vi "main.vi"() -> ()   [LabVIEW 2018]
uses:
  controls/Button Previous.ctl
  controls/Button Next.ctl
  support/classes/MonthDisplay/month.ctl
  support/classes/Banking Statement/BankingTransactionList.lvclass
  C:/GitRepos/Filthy-Lucre-Budgetizer/source/support/classes/Statement/TransactionList.lvclass
  support/classes/Credit Statement/CreditTransactionList.lvclass
  support/classes/Goal/Goal.lvclass
  C:/GitRepos/Filthy-Lucre-Budgetizer/source/support/classes/UserEditableAmount/UserEditableAmount.lvclass
  support/classes/TransactionListUserInterface/TransactionListUIAdapter.lvclass
  support/classes/database/Account History.lvclass
  support/classes/UserEditableAmount/UserEditableAmount.lvclass
  support/classes/Category/Category.lvclass
  support/classes/MonthDisplay/DateUserInterface.lvclass
  support/classes/GoalUserInterface/OutcomeListUIAdapter.lvclass
panel:
  in  "Month":T1
  in  "Tab Control":enum32{"Summary", "Banking", "Credit", "Report"}(tab)
  in  "Delete Goal":bool
  in  "Edit Goal":bool
  in  "Summary":i32(listbox)
  out "Banking":i32(listbox)
  in  "Credit":i32[](listbox)
  out "Balance":dbl format="%.2f"
  in  "Next":T2
  in  "Prev":T3
  in  "Year":i32=2008
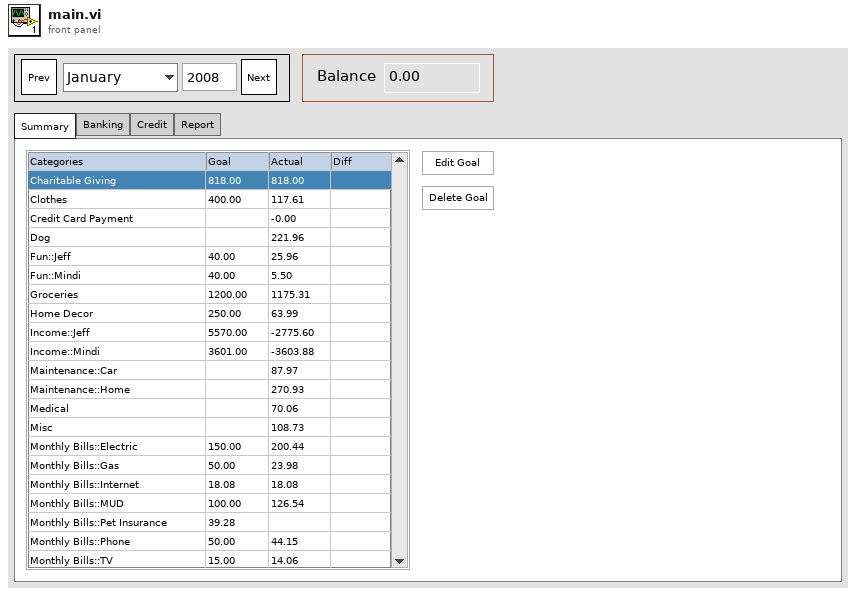
[diagram p1: front panel]
types:
  T1 = typedef "DateUserInterface.lvclass/month.ctl" = enum16{"January", "February", "March", "April", "May", "June", "July", "August", "September", "October", "November", "December"}
  T2 = typedef "Button Next.ctl" = bool
  T3 = typedef "Button Previous.ctl" = bool
  T4 = enum8{"Enabled", "Disabled", "Disabled and Grayed Out"}
  T5 = typedef "LVPoint32TypeDef.ctl" = cluster{"Horizontal":i32, "Vertical":i32}
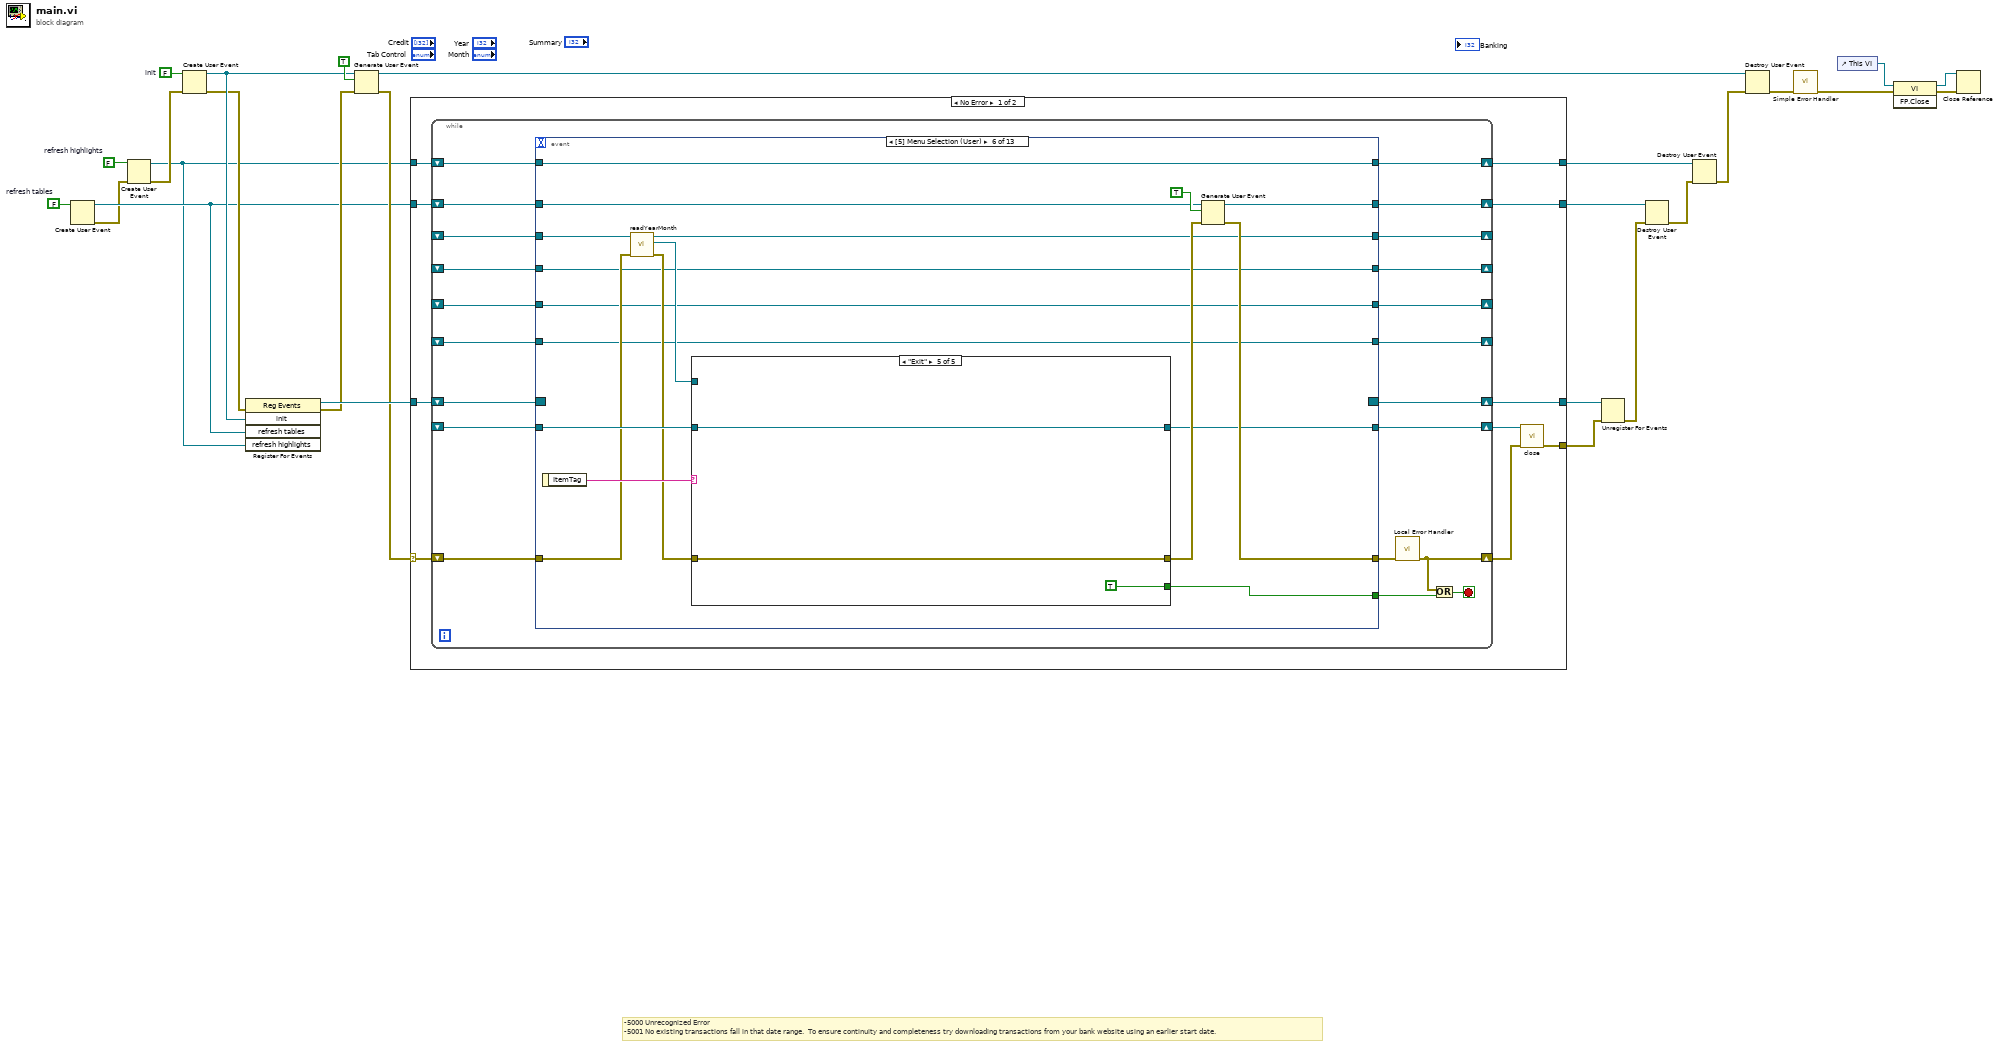
[diagram p0: block diagram]
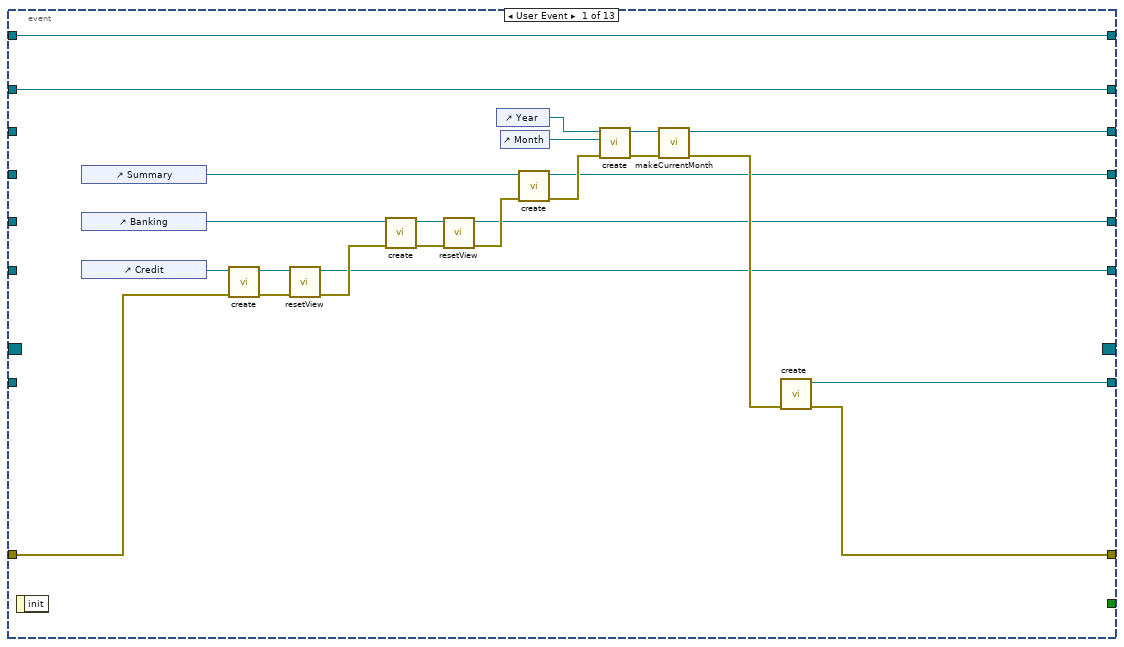
[diagram p2: hidden frame]
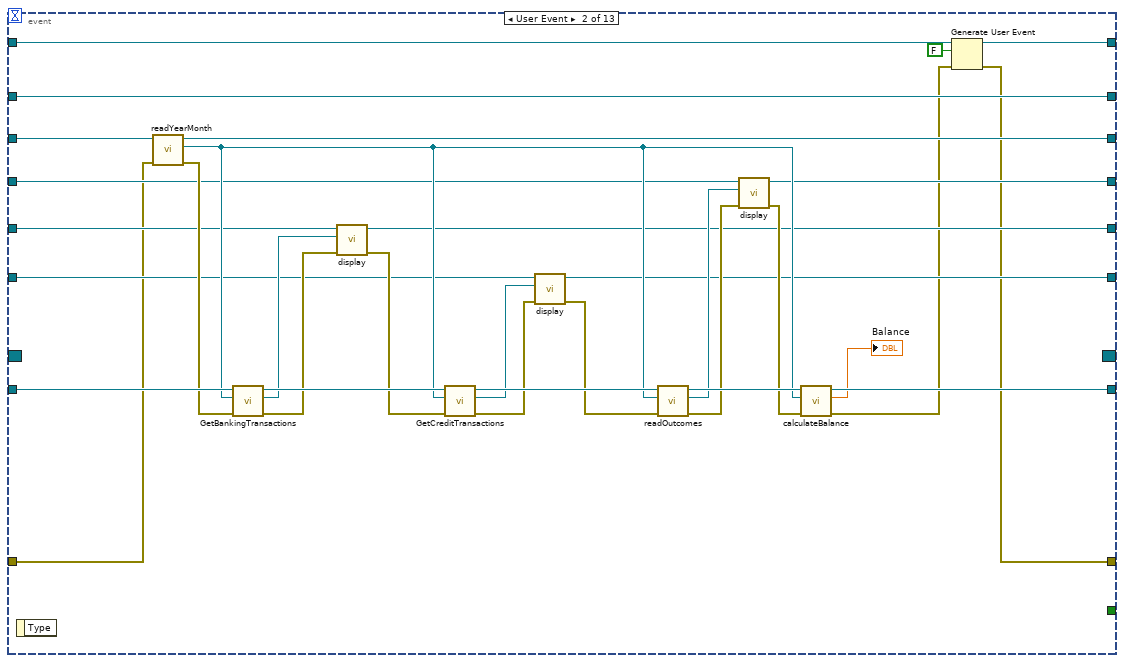
[diagram p3: hidden frame]
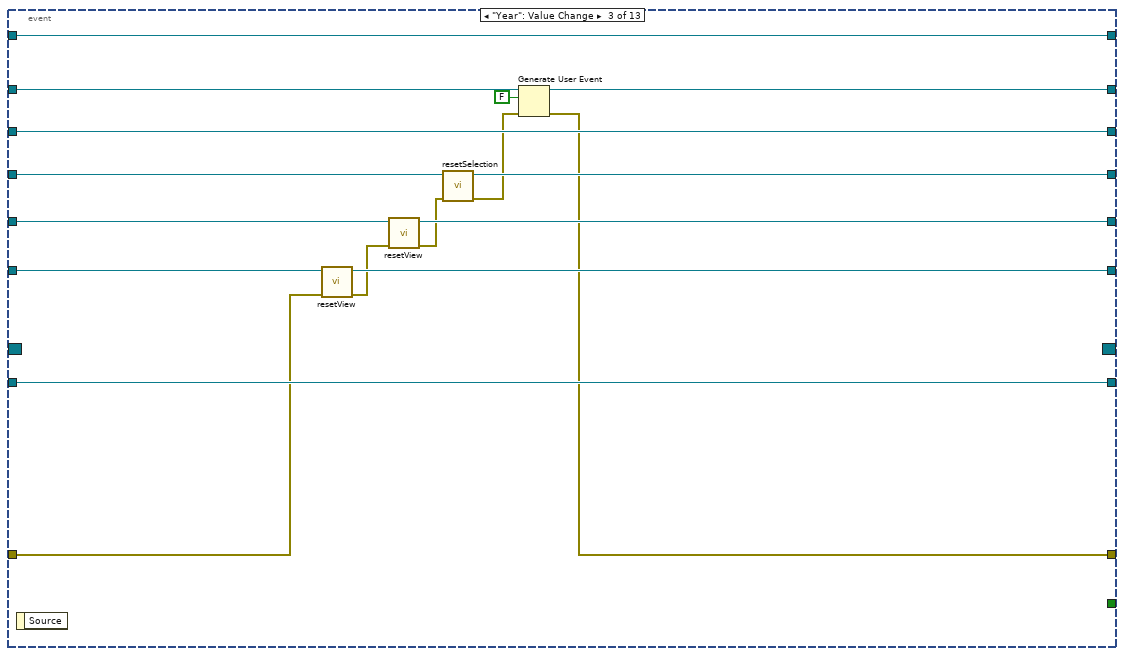
[diagram p4: hidden frame]
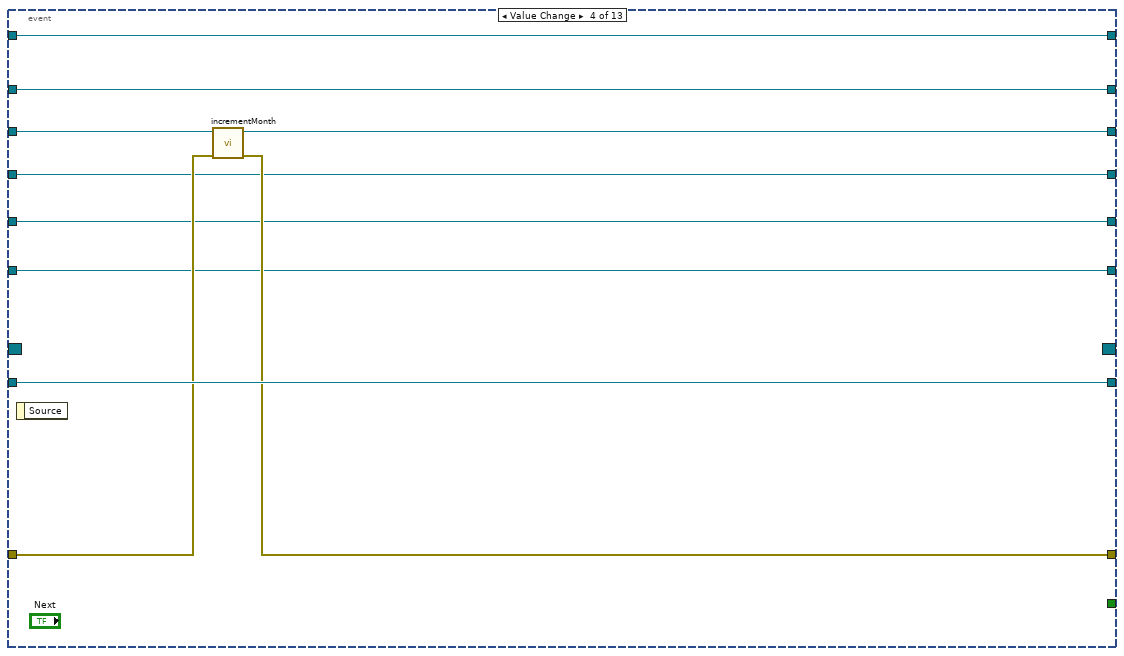
[diagram p5: hidden frame]
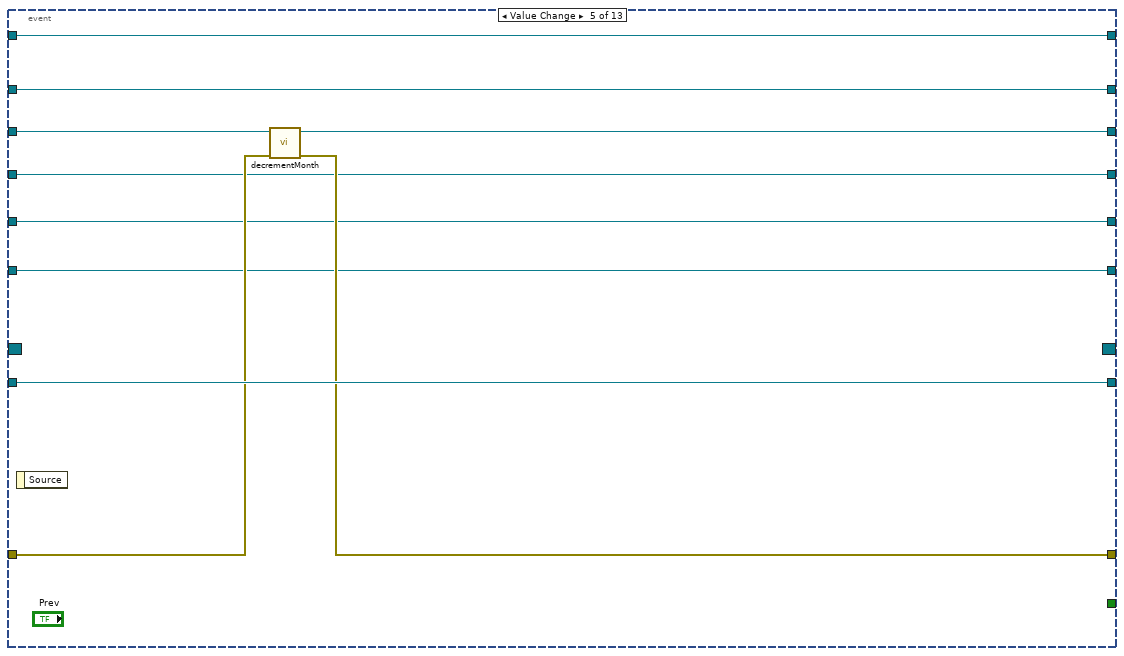
[diagram p6: hidden frame]
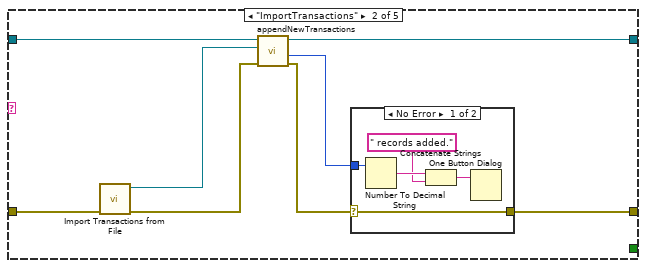
[diagram p8: hidden frame]
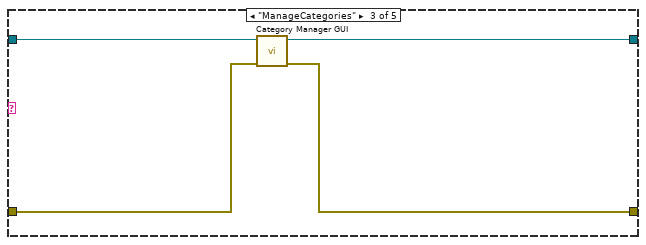
[diagram p10: hidden frame]
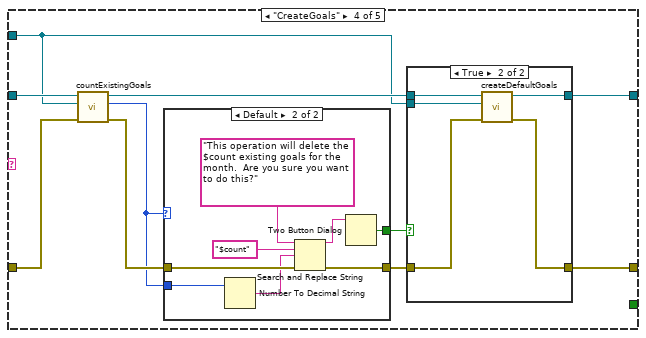
[diagram p11: hidden frame]
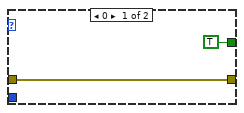
[diagram p12: hidden frame]
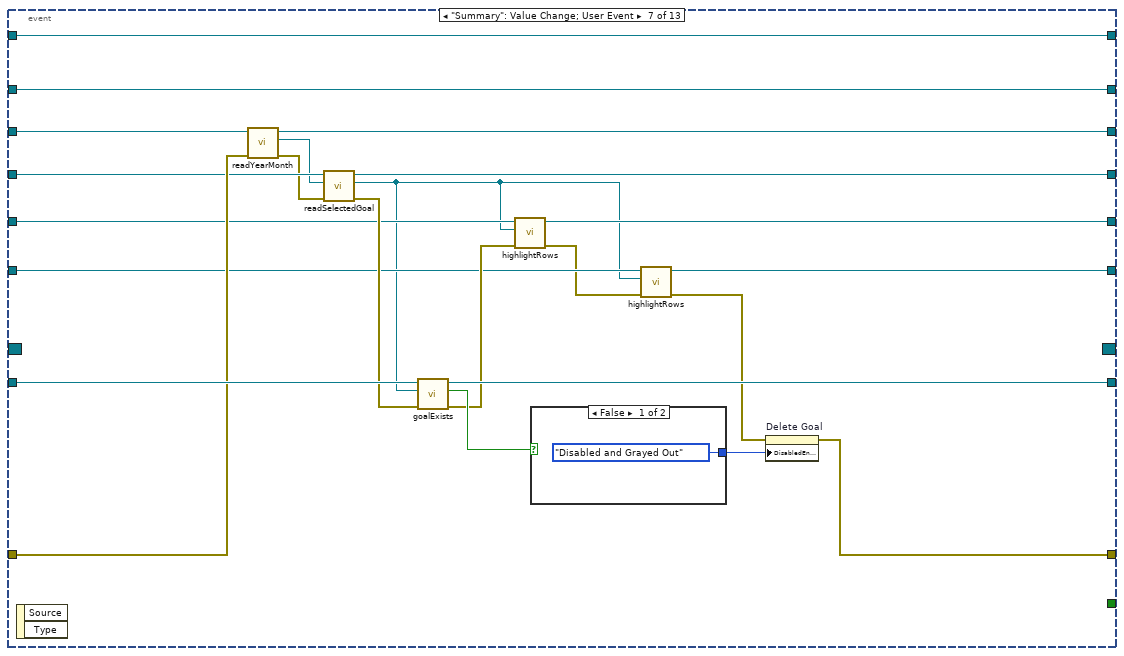
[diagram p14: hidden frame]
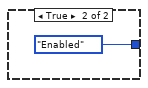
[diagram p15: hidden frame]
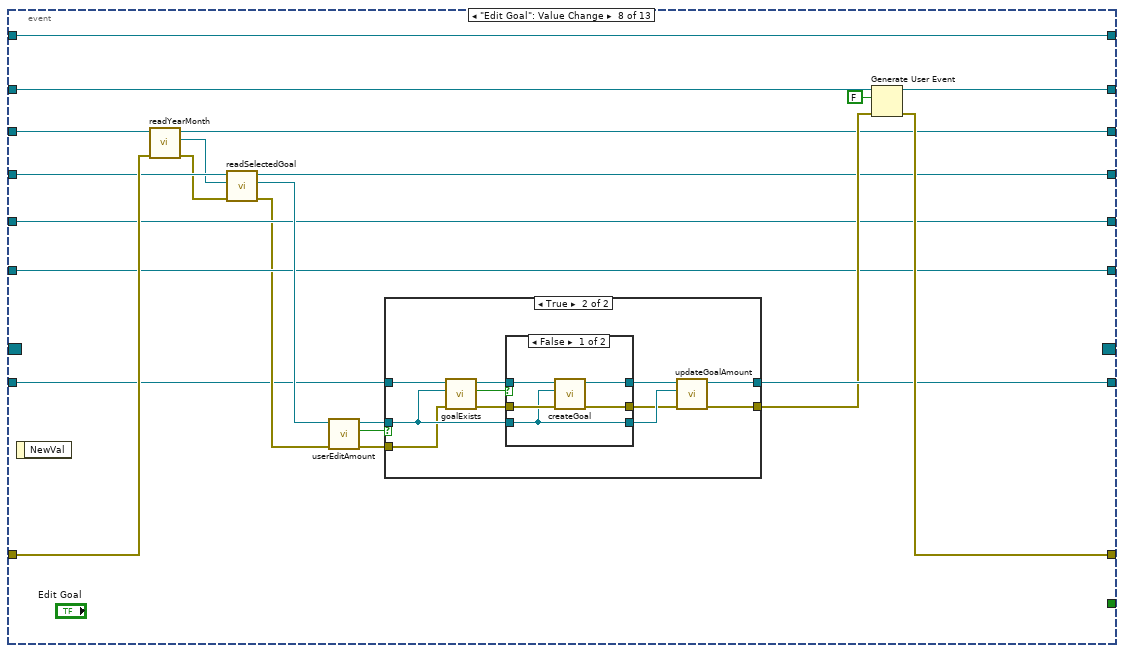
[diagram p16: hidden frame]
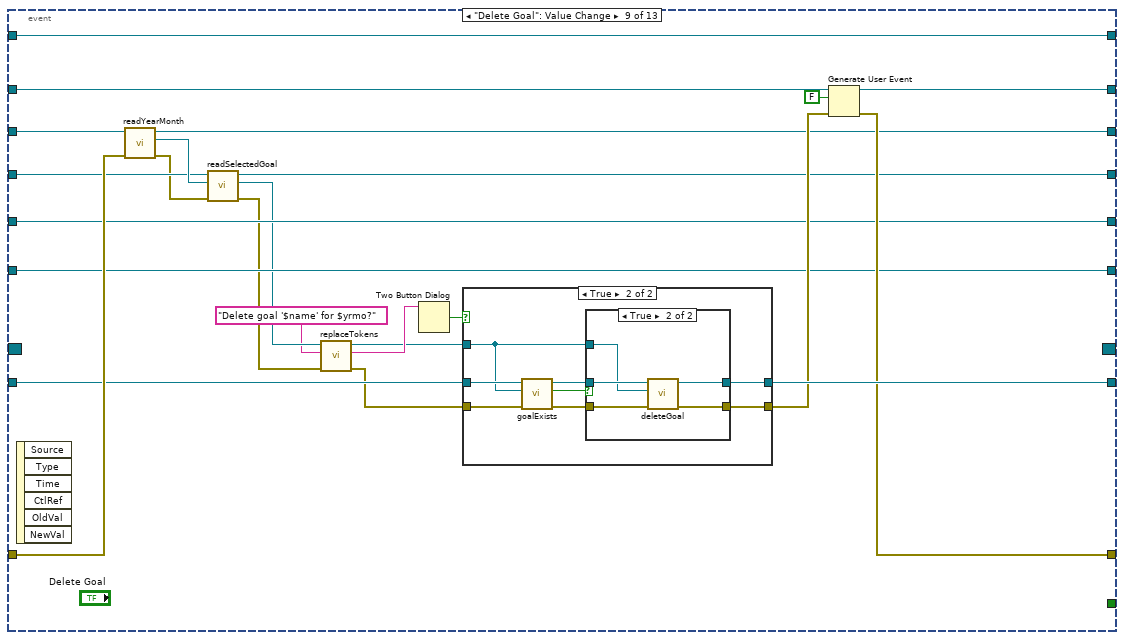
[diagram p19: hidden frame]
diagram:
  w5 = FALSE  # refresh highlights
  w15 = FALSE  # refresh tables
  w24 = FALSE  # init
  # "-5000 Unrecognized Error\n-5001 No existing transactions fall in that date range.  To ensure continuity and completeness try downloading transactions from your bank website using an earlier start date."
  n1 = Create User Event(user event datatype=w15) -> (user event=w14:refnum<user-event>, error out=w7:errorcluster)  [unwired: 1 in]
  n2 = Create User Event(user event datatype=w5, error in=w7) -> (user event=w4:refnum<user-event>, error out=w6:errorcluster)
  n3 = Create User Event(user event datatype=w24, error in=w6) -> (user event=w21:refnum<user-event>, error out=w17:errorcluster)
  n4 = register-events(error in=w17, w21, w14, w4) -> (reference out=w26:refnum<event-registration>, error out=w20:errorcluster)  [unwired: 1 in]
  n5 = Generate User Event(user event=w21, event data cluster=TRUE ("event data"), error in=w20) -> (user event out=w18:refnum<user-event>, error out=w19:errorcluster)  [unwired: 1 in]
  n6 = case shown="No Error" w19 {
    selector: w19 -> [w34 w396]
    tunnel: w26 -> [w36 w397]
    tunnel: [w29 w396] -> w16
    tunnel: [w35 w397] -> w25
    tunnel: w14 -> [w33 w395]
    tunnel: [w32 w395] -> w13
    tunnel: w4 -> [w28 w394]
    tunnel: [w27 w394] -> w3
    frame No Error {
      n7 = while {
        shift-right: [w53] -> w30
        shift-left: w34 -> [w56]
        shift-right: [w55] -> w35
        shift-left: w36 -> [w57]
        shift-right: [w49] -> w31
        shift-left: _ -> [w50]
        shift-right: [w47] -> w32
        shift-left: w33 -> [w48]
        shift-right: [w46] -> _
        shift-left: _ -> [w43]
        shift-right: [w45] -> _
        shift-left: _ -> [w44]
        shift-right: [w42] -> _
        shift-left: _ -> [w41]
        shift-right: [w40] -> _
        shift-left: _ -> [w39]
        shift-right: [w37] -> w27
        shift-left: w28 -> [w38]
        stop <- w52 stop-if-true
        n8 = event shown="[5] Menu Selection (User)" {
          selector: w57 -> [_ _ _ _ _ _ _ _ _ _ _ _ _]
          dyn-events: [_ _ _ _ _ _ _ _ _ _ _ _ _] -> w55
          timeout: _ -> [_ _ _ _ _ _ _ _ _ _ _ _ _]
          tunnel: w56 -> [w67 w87 w119 w137 w146 w157 w234 w258 w304 w335 w356 w366 w393]
          tunnel: [w79 w83 w114 w135 w145 w163 w238 w263 w307 w346 w355 w382 w393] -> w54
          tunnel: [_ _ _ _ _ w151 _ _ _ _ _ _ w386] -> w51
          tunnel: w50 -> [_ w112 w128 w140 w150 w167 w240 w244 w302 w341 w360 w380 w391]
          tunnel: [w81 w111 w128 w140 w150 w161 w239 w262 w310 w341 w359 w379 w391] -> w49
          tunnel: w48 -> [w80 w113 w130 w139 w149 w165 w241 w265 w308 w342 w354 w383 w392]
          tunnel: [w80 w113 w129 w139 w149 w164 w241 w264 w309 w342 w354 w384 w392] -> w47
          tunnel: [w75 w106 w127 w136 w147 w159 w233 w259 w303 w332 w352 w377 w390] -> w46
          tunnel: w43 -> [_ w107 w127 w138 w148 w160 w235 w260 w305 w332 w352 w377 w390]
          tunnel: [w70 w99 w121 w134 w144 w155 w231 w251 w298 w331 w351 w376 w389] -> w45
          tunnel: w44 -> [_ w88 w120 w134 w144 w155 w232 w254 w300 w331 w351 w376 w389]
          tunnel: [w62 w98 w123 w133 w143 w154 w225 w249 w296 w330 w350 w374 w388] -> w42
          tunnel: w41 -> [_ w90 w125 w133 w143 w154 w227 w249 w296 w330 w350 w374 w388]
          tunnel: [w58 w91 w122 w132 w142 w153 w221 w248 w297 w329 w349 w373 w387] -> w40
          tunnel: w39 -> [_ w89 w124 w132 w142 w153 w224 w248 w297 w329 w349 w373 w387]
          tunnel: w38 -> [w66 w86 w115 w131 w141 w152 w219 w246 w294 w328 w348 w363 w385]
          tunnel: [w66 w85 w115 w131 w141 w152 w219 w246 w294 w328 w348 w363 w385] -> w37
          event User Event {
            n9 = event-data() -> ()  [unwired: 1 in, 1 out]
            n10 = control-ref of="Summary"() -> (w73:refnum<vi>)
            n11 = control-ref of="Banking"() -> (w69:refnum<vi>)
            n12 = control-ref of="Credit"() -> (w68:refnum<vi>)
            n13 = call "create.vi"("error in (no error)"=w67, "MulticolumnListbox in"=w68) -> ("error out"=w61:errorcluster, "TransactionListUserInterface out"=w60:refnum<class "TransactionListUIAdapter.lvclass">)  [unwired: 8 in]
            n14 = call-dynamic "resetView.vi"("error in (no error)"=w61, "TransactionListUserInterface in"=w60) -> ("error out"=w59:errorcluster, "TransactionListUserInterface out"=w58:refnum<class "TransactionListUIAdapter.lvclass">)  [unwired: 8 in]
            n15 = call "create.vi"("error in (no error)"=w59, "MulticolumnListbox in"=w69) -> ("error out"=w64:errorcluster, "TransactionListUserInterface out"=w65:refnum<class "TransactionListUIAdapter.lvclass">)  [unwired: 8 in]
            n16 = call-dynamic "resetView.vi"("error in (no error)"=w64, "TransactionListUserInterface in"=w65) -> ("error out"=w63:errorcluster, "TransactionListUserInterface out"=w62:refnum<class "TransactionListUIAdapter.lvclass">)  [unwired: 8 in]
            n17 = control-ref of="Year"() -> (w78:refnum<vi>)
            n18 = control-ref of="Month"() -> (w77:refnum<vi>)
            n19 = call "create.vi"("error in (no error)"=w63, "Summary"=w73) -> ("error out"=w71:errorcluster, "GoalUserInterface out"=w70:refnum<class "OutcomeListUIAdapter.lvclass">)  [unwired: 8 in]
            n20 = call "create.vi"("error in (no error)"=w71, "Month"=w77, "Year"=w78) -> ("error out"=w74:errorcluster, "MonthDisplay out"=w76:refnum<class "DateUserInterface.lvclass">)  [unwired: 7 in]
            n21 = call "makeCurrentMonth.vi"("error in (no error)"=w74, "MonthDisplay in"=w76) -> ("error out"=w72:errorcluster, "MonthDisplay out"=w75:refnum<class "DateUserInterface.lvclass">)  [unwired: 8 in]
            n22 = call "create.vi"("error in (no error)"=w72) -> ("error out"=w79:errorcluster, "Database.lvclass"=w81:refnum<class "Account History.lvclass">)  [unwired: 9 in]
          }
          event User Event {
            n23 = event-data() -> ()  [unwired: 1 in, 1 out]
            n24 = call "readYearMonth.vi"("error in (no error)"=w87, "MonthDisplay in"=w107) -> ("error out"=w104:errorcluster, "WhichMonth.lvclass"=w105:refnum<class "WhichMonth.lvclass">, "MonthDisplay out"=w106:refnum<class "DateUserInterface.lvclass">)  [unwired: 7 in]
            n25 = call "GetBankingTransactions.vi"("error in (no error)"=w104, "WhichMonth"=w105, "Database in"=w112) -> ("error out"=w96:errorcluster, "Banking Transactions out"=w97:refnum<class "BankingTransactionList.lvclass">, "Database out"=w109:refnum<class "Account History.lvclass">)  [unwired: 6 in]
            n26 = call "display.vi"("error in (no error)"=w96, "TransactionList.lvclass"=w97, "TransactionListUserInterface in"=w90) -> ("error out"=w95:errorcluster, "TransactionListUserInterface out"=w98:refnum<class "TransactionListUIAdapter.lvclass">)  [unwired: 7 in]
            n27 = call "GetCreditTransactions.vi"("error in (no error)"=w95, "WhichMonth"=w105, "Account History in"=w109) -> ("error out"=w93:errorcluster, "Credit Transactions out"=w94:refnum<class "CreditTransactionList.lvclass">, "Account History out"=w108:refnum<class "Account History.lvclass">)  [unwired: 6 in]
            n28 = call "display.vi"("error in (no error)"=w93, "TransactionList.lvclass"=w94, "TransactionListUserInterface in"=w89) -> ("error out"=w92:errorcluster, "TransactionListUserInterface out"=w91:refnum<class "TransactionListUIAdapter.lvclass">)  [unwired: 7 in]
            n29 = call "readOutcomes.vi"("error in (no error)"=w92, "WhichMonth"=w105, "Database in"=w108) -> ("error out"=w102:errorcluster, "OutcomeList.lvclass"=w103:refnum<class "OutcomeList.lvclass">, "Database out"=w110:refnum<class "Account History.lvclass">)  [unwired: 6 in]
            n30 = call "display.vi"("error in (no error)"=w102, "OutcomeList.lvclass"=w103, "GoalUserInterface in"=w88) -> ("error out"=w101:errorcluster, "GoalUserInterface out"=w99:refnum<class "OutcomeListUIAdapter.lvclass">)  [unwired: 7 in]
            n31 = call "calculateBalance.vi"("error in (no error)"=w101, "WhichMonth"=w105, "Database in"=w110) -> ("error out"=w84:errorcluster, "Month Balance"=→"Balance":dbl, "Database out"=w111:refnum<class "Account History.lvclass">)  [unwired: 6 in]
            n32 = Generate User Event(user event=w86, event data cluster=FALSE ("event data"), error in=w84) -> (user event out=w85:refnum<user-event>, error out=w83:errorcluster)  [unwired: 1 in]
          }
          event "Year": Value Change {
            n33 = event-data() -> ()  [unwired: 1 in, 1 out]
            n34 = call-dynamic "resetView.vi"("error in (no error)"=w119, "TransactionListUserInterface in"=w124) -> ("error out"=w118:errorcluster, "TransactionListUserInterface out"=w122:refnum<class "TransactionListUIAdapter.lvclass">)  [unwired: 8 in]
            n35 = call-dynamic "resetView.vi"("error in (no error)"=w118, "TransactionListUserInterface in"=w125) -> ("error out"=w117:errorcluster, "TransactionListUserInterface out"=w123:refnum<class "TransactionListUIAdapter.lvclass">)  [unwired: 8 in]
            n36 = call "resetSelection.vi"("error in (no error)"=w117, "GoalUserInterface in"=w120) -> ("error out"=w116:errorcluster, "GoalUserInterface out"=w121:refnum<class "OutcomeListUIAdapter.lvclass">)  [unwired: 8 in]
            n37 = Generate User Event(user event=w130, event data cluster=FALSE ("event data"), error in=w116) -> (user event out=w129:refnum<user-event>, error out=w114:errorcluster)  [unwired: 1 in]
          }
          event Value Change {
            n38 = event-data() -> ()  [unwired: 1 in, 1 out]
            n39 = call "incrementMonth.vi"("error in (no error)"=w137, "MonthDisplay in"=w138) -> ("error out"=w135:errorcluster, "MonthDisplay out"=w136:refnum<class "DateUserInterface.lvclass">)  [unwired: 8 in]
          }
          event Value Change {
            n40 = event-data() -> ()  [unwired: 1 in, 1 out]
            n41 = call "decrementMonth.vi"("error in (no error)"=w146, "MonthDisplay in"=w148) -> ("error out"=w145:errorcluster, "MonthDisplay out"=w147:refnum<class "DateUserInterface.lvclass">)  [unwired: 8 in]
          }
          event Menu Selection (User) {
            n42 = event-data() -> ("ItemTag"=w168:string)  [unwired: 1 in]
            n43 = call "readYearMonth.vi"("error in (no error)"=w157, "MonthDisplay in"=w160) -> ("error out"=w156:errorcluster, "WhichMonth.lvclass"=w158:refnum<class "WhichMonth.lvclass">, "MonthDisplay out"=w159:refnum<class "DateUserInterface.lvclass">)  [unwired: 7 in]
            n44 = case shown="\"Exit\"" w168 {
              tunnel: w156 -> [w170 w178 w186 w193 w217]
              tunnel: [w170 w174 w185 w197 w217] -> w162
              tunnel: w167 -> [w169 w177 w188 w196 w218]
              tunnel: [w169 w176 w187 w198 w218] -> w161
              tunnel: w158 -> [_ _ _ w194 _]
              tunnel: [_ _ _ _ TRUE] -> w151
              frame Default {
              }
              frame "ImportTransactions" {
                n45 = call "Import Transactions from File.vi"("error in (no error)"=w178) -> ("error out"=w173:errorcluster, "Importing Statement"=w172:refnum<class "TransactionList.lvclass">)  [unwired: 9 in]
                n46 = call "appendNewTransactions.vi"("error in (no error)"=w173, "TransactionList.lvclass"=w172, "Database in"=w177) -> ("error out"=w175:errorcluster, "Num records"=w171:i32, "Database out"=w176:refnum<class "Account History.lvclass">)  [unwired: 6 in]
                n47 = case shown="No Error" w175 {
                  selector: w175 -> [w180 w184]
                  tunnel: [w180 w184] -> w174
                  tunnel: w171 -> [w179 _]
                  frame No Error {
                    n48 = Number To Decimal String(number=w179) -> (decimal integer string=w182:string)  [unwired: 1 in]
                    n49 = Concatenate Strings(w182, " records added.") -> (w183:string)
                    n50 = One Button Dialog(message=w183) -> ()  [unwired: 1 in, 1 out]
                  }
                  frame Error {
                  }
                }
              }
              frame "ManageCategories" {
                n51 = call "Category Manager GUI.vi"("error in (no error)"=w186, "Database.lvclass"=w188) -> ("error out"=w185:errorcluster, "Database.lvclass"=w187:refnum<class "Account History.lvclass">)  [unwired: 8 in]
              }
              frame "CreateGoals" {
                n52 = call "countExistingGoals.vi"("error in (no error)"=w193, "WhichMonth.lvclass"=w194, "Account History in"=w196) -> ("error out"=w192:errorcluster, "Goal  Count"=w189:i32, "Account History out"=w195:refnum<class "Account History.lvclass">)  [unwired: 6 in]
                n53 = case shown="Default" w189 {
                  tunnel: w192 -> [w200 w208]
                  tunnel: w189 -> [_ w207]
                  tunnel: [TRUE ("T button?") w206] -> w191
                  tunnel: [w200 w205] -> w190
                  frame 0 {
                  }
                  frame Default {
                    n54 = Number To Decimal String(number=w207) -> (decimal integer string=w201:string)  [unwired: 1 in]
                    n55 = Search and Replace String(input string="This operation will delete the $count existing goals for the month.  Are you sure you want to do this?", search string="$count", replace string=w201, error in=w208) -> (result string=w204:string, error out=w205:errorcluster)  [unwired: 4 in, 2 out]
                    n56 = Two Button Dialog(message=w204) -> (T button?=w206:bool)  [unwired: 2 in]
                  }
                }
                n57 = case shown="True" w191 {
                  tunnel: w195 -> [w210 w215]
                  tunnel: [w210 w214] -> w198
                  tunnel: w190 -> [w209 w213]
                  tunnel: [w209 w212] -> w197
                  tunnel: w194 -> [_ w211]
                  frame False {
                  }
                  frame True {
                    n58 = call "createDefaultGoals.vi"("error in (no error)"=w213, "WhichMonth"=w211, "Database in"=w215) -> ("error out"=w212:errorcluster, "Database out"=w214:refnum<class "Account History.lvclass">)  [unwired: 7 in]
                  }
                }
              }
              frame "Exit" {
              }
            }
            n59 = Generate User Event(user event=w165, event data cluster=TRUE ("event data"), error in=w162) -> (user event out=w164:refnum<user-event>, error out=w163:errorcluster)  [unwired: 1 in]
          }
          event "Summary": Value Change; User Event {
            n60 = event-data() -> ()  [unwired: 1 in, 2 out]
            n61 = call "readYearMonth.vi"("error in (no error)"=w234, "MonthDisplay in"=w235) -> ("error out"=w230:errorcluster, "WhichMonth.lvclass"=w229:refnum<class "WhichMonth.lvclass">, "MonthDisplay out"=w233:refnum<class "DateUserInterface.lvclass">)  [unwired: 7 in]
            n62 = call "readSelectedGoal.vi"("error in (no error)"=w230, "WhichMonth.lvclass"=w229, "GoalUserInterface in"=w232) -> ("error out"=w228:errorcluster, "Goal.lvclass"=w223:refnum<class "Goal.lvclass">, "GoalUserInterface out"=w231:refnum<class "OutcomeListUIAdapter.lvclass">)  [unwired: 6 in]
            n63 = call "goalExists.vi"("error in (no error)"=w228, "Goal.lvclass"=w223, "Account History in"=w240) -> ("error out"=w226:errorcluster, "Exists?"=w237:bool, "Account History out"=w239:refnum<class "Account History.lvclass">)  [unwired: 6 in]
            n64 = call "highlightRows.vi"("error in (no error)"=w226, "Goal.lvclass"=w223, "TransactionListUserInterface in"=w227) -> ("error out"=w222:errorcluster, "TransactionListUserInterface out"=w225:refnum<class "TransactionListUIAdapter.lvclass">)  [unwired: 7 in]
            n65 = case shown="False" w237 {
              tunnel: [T4."Disabled and Grayed Out" ("Disabled") T4."Enabled" ("Disabled")] -> w236
              frame False {
              }
              frame True {
              }
            }
            n66 = call "highlightRows.vi"("error in (no error)"=w222, "Goal.lvclass"=w223, "TransactionListUserInterface in"=w224) -> ("error out"=w220:errorcluster, "TransactionListUserInterface out"=w221:refnum<class "TransactionListUIAdapter.lvclass">)  [unwired: 7 in]
            n67 = property on="Delete Goal" class="Bool"(error in=w220, "DisabledEnum"=w236) -> (error out=w238:errorcluster)  [unwired: 1 in, 1 out]
          }
          event "Edit Goal": Value Change {
            n68 = event-data() -> ()  [unwired: 1 in, 1 out]
            n69 = call "readYearMonth.vi"("error in (no error)"=w258, "MonthDisplay in"=w260) -> ("error out"=w252:errorcluster, "WhichMonth.lvclass"=w253:refnum<class "WhichMonth.lvclass">, "MonthDisplay out"=w259:refnum<class "DateUserInterface.lvclass">)  [unwired: 7 in]
            n70 = call "readSelectedGoal.vi"("error in (no error)"=w252, "WhichMonth.lvclass"=w253, "GoalUserInterface in"=w254) -> ("error out"=w245:errorcluster, "Goal.lvclass"=w250:refnum<class "Goal.lvclass">, "GoalUserInterface out"=w251:refnum<class "OutcomeListUIAdapter.lvclass">)  [unwired: 6 in]
            n71 = call "userEditAmount.vi"("error in (no error)"=w245, "UserEditableAmount.lvclass"=w250) -> ("error out"=w256:errorcluster, "UserConfirm?"=w255:bool, "UserEditableAmount.lvclass"=w257:refnum<class "Goal.lvclass">)  [unwired: 7 in]
            n72 = case shown="True" w255 {
              tunnel: w257 -> [_ w271]
              tunnel: w256 -> [w266 w270]
              tunnel: w244 -> [w267 w273]
              tunnel: [w267 w278] -> w262
              tunnel: [w266 w277] -> w261
              frame False {
              }
              frame True {
                n73 = call "goalExists.vi"("error in (no error)"=w270, "Goal.lvclass"=w271, "Account History in"=w273) -> ("error out"=w275:errorcluster, "Exists?"=w276:bool, "Account History out"=w274:refnum<class "Account History.lvclass">)  [unwired: 6 in]
                n74 = case shown="False" w276 {
                  tunnel: w274 -> [w283 w286]
                  tunnel: w275 -> [w282 w285]
                  tunnel: [w281 w285] -> w268
                  tunnel: [w280 w286] -> w272
                  tunnel: w271 -> [w279 w284]
                  tunnel: [w279 w284] -> w269
                  frame False {
                    n75 = call "createGoal.vi"("error in (no error)"=w282, "Goal.lvclass"=w279, "Account History in"=w283) -> ("error out"=w281:errorcluster, "Account History out"=w280:refnum<class "Account History.lvclass">)  [unwired: 7 in]
                  }
                  frame True {
                  }
                }
                n76 = call "updateGoalAmount.vi"("error in (no error)"=w268, "Goal.lvclass"=w269, "Database in"=w272) -> ("error out"=w277:errorcluster, "Database out"=w278:refnum<class "Account History.lvclass">)  [unwired: 7 in]
              }
            }
            n77 = Generate User Event(user event=w265, event data cluster=FALSE ("event data"), error in=w261) -> (user event out=w264:refnum<user-event>, error out=w263:errorcluster)  [unwired: 1 in]
          }
          event "Delete Goal": Value Change {
            n78 = event-data() -> ()  [unwired: 1 in, 6 out]
            n79 = call "readYearMonth.vi"("error in (no error)"=w304, "MonthDisplay in"=w305) -> ("error out"=w299:errorcluster, "WhichMonth.lvclass"=w301:refnum<class "WhichMonth.lvclass">, "MonthDisplay out"=w303:refnum<class "DateUserInterface.lvclass">)  [unwired: 7 in]
            n80 = call "readSelectedGoal.vi"("error in (no error)"=w299, "WhichMonth.lvclass"=w301, "GoalUserInterface in"=w300) -> ("error out"=w292:errorcluster, "Goal.lvclass"=w293:refnum<class "Goal.lvclass">, "GoalUserInterface out"=w298:refnum<class "OutcomeListUIAdapter.lvclass">)  [unwired: 6 in]
            n81 = call "replaceTokens.vi"("error in (no error)"=w292, "Querry In"="Delete goal '$name' for $yrmo?", "Goal in"=w293) -> ("error out"=w288:errorcluster, "Query Out"=w290:string, "Goal out"=w289:refnum<class "Goal.lvclass">)  [unwired: 6 in]
            n82 = Two Button Dialog(message=w290) -> (T button?=w287:bool)  [unwired: 2 in]
            n83 = case shown="True" w287 {
              tunnel: [w312 w320] -> w310
              tunnel: [w311 w319] -> w306
              tunnel: w302 -> [w312 w315]
              tunnel: w288 -> [w311 w314]
              tunnel: w289 -> [_ w313]
              frame False {
              }
              frame True {
                n84 = call "goalExists.vi"("error in (no error)"=w314, "Goal.lvclass"=w313, "Account History in"=w315) -> ("error out"=w317:errorcluster, "Exists?"=w316:bool, "Account History out"=w318:refnum<class "Account History.lvclass">)  [unwired: 6 in]
                n85 = case shown="True" w316 {
                  tunnel: w318 -> [w322 w327]
                  tunnel: w317 -> [w321 w326]
                  tunnel: [w322 w325] -> w320
                  tunnel: [w321 w324] -> w319
                  tunnel: w313 -> [_ w323]
                  frame False {
                  }
                  frame True {
                    n86 = call "deleteGoal.vi"("error in (no error)"=w326, "Goal.lvclass"=w323, "Account History in"=w327) -> ("error out"=w324:errorcluster, "Account History out"=w325:refnum<class "Account History.lvclass">)  [unwired: 7 in]
                  }
                }
              }
            }
            n87 = Generate User Event(user event=w308, event data cluster=FALSE ("event data"), error in=w306) -> (user event out=w309:refnum<user-event>, error out=w307:errorcluster)  [unwired: 1 in]
          }
          event "Banking", "Credit": Mouse Down? {
            # "Right Mouse Button"
            n88 = event-data() -> ("CtlRef"=w334:refnum<vi>, "Coords"=w347:T5)  [unwired: 1 in]
            n89 = call "Find Table Cell from Coordinate.vi"("error in (no error)"=w335, "Coords"=w347, "MCLB Refs"=w334) -> ("error out"=w346:errorcluster, "Found?"=w333:bool, "Column"=w343:u32)  [unwired: 5 in, 1 out]
            n90 = Equal?(x=u32 3, y=w343) -> (x = y?=w344:bool)
            n91 = Compound Arithmetic op=AND(w344, w333) -> (w339:bool)
            n92 = Select(t=u16 2 ("Button"), s=w339, f=u16 1) -> (s? t:f=w336:u16)
            n93 = event-data("Button"=w336, "Discard?"=FALSE) -> ()  [unwired: 1 in, 1 out]
          }
          event "Banking", "Credit": Shortcut Menu Activation? {
            n94 = event-data() -> ("MenuRef"=w358:refnum<k9>)  [unwired: 1 in]
            n95 = call "getCategoriesLikeName.vi"("error in (no error)"=w356, "Name filter"="", "Database in"=w360) -> ("error out"=w357:errorcluster, "CategoryList out"=w353:refnum<class "CategoryList.lvclass">, "Database out"=w359:refnum<class "Account History.lvclass">)  [unwired: 6 in]
            n96 = call "Construct Category Menu.vi"("error in (no error)"=w357, "CategoryList.lvclass"=w353, "Menu in"=w358) -> ("error out"=w355:errorcluster)  [unwired: 8 in]
            n97 = event-data("Discard?"=FALSE) -> ()  [unwired: 1 in, 1 out]
          }
          event "Banking", "Credit": Shortcut Menu Selection (User) {
            n98 = event-data() -> ("ItemTag"=w375:string, "CtlRef"=w372:refnum<vi>, "Coords"=w369:T5)  [unwired: 1 in]
            n99 = call "create.vi"("error in (no error)"=w366, "Name"=w375) -> ("error out"=w365:errorcluster, "Category out"=w381:refnum<class "Category.lvclass">)  [unwired: 8 in]
            n100 = call "create.vi"("error in (no error)"=w365, "MulticolumnListbox in"=w372) -> ("error out"=w370:errorcluster, "TransactionListUserInterface out"=w371:refnum<class "TransactionListUIAdapter.lvclass">)  [unwired: 8 in]
            n101 = call "findTransactionClicked.vi"("error in (no error)"=w370, "Coords"=w369, "TransactionListUserInterface in"=w371) -> ("error out"=w368:errorcluster, "Transaction.lvclass"=w367:refnum<class "Transaction.lvclass">)  [unwired: 6 in, 1 out]
            n102 = call "setTransactionCategory.vi"("error in (no error)"=w368, "Transaction"=w367, "Category.lvclass"=w381, "Database in"=w380) -> ("error out"=w378:errorcluster, "Database out"=w379:refnum<class "Account History.lvclass">)  [unwired: 6 in]
            n103 = Generate User Event(user event=w383, event data cluster=FALSE ("event data"), error in=w378) -> (user event out=w384:refnum<user-event>, error out=w382:errorcluster)  [unwired: 1 in]
          }
          event Panel Close? {
            w386 = TRUE ("Discard?")
            n104 = event-data() -> ()  [unwired: 1 in, 1 out]
            n105 = event-data("Discard?"=w386) -> ()  [unwired: 1 in, 1 out]
          }
        }
        n106 = call "Local Error Handler.vi"("error in"=w54) -> ("error out"=w53:errorcluster)  [unwired: 10 in]
        n107 = Or(x=w53, y=w51) -> (x .or. y?=w52:bool)
      }
      n108 = call "close.vi"("error in (no error)"=w30, "Database.lvclass"=w31) -> ("error out"=w29:errorcluster)  [unwired: 9 in]
    }
    frame Error {
    }
  }
  n109 = Unregister For Events(event registration refnum=w25, error in=w16) -> (error out=w12:errorcluster)
  n110 = Destroy User Event(user event=w13, error in=w12) -> (error out=w2:errorcluster)
  n111 = Destroy User Event(user event=w3, error in=w2) -> (error out=w1:errorcluster)
  n112 = Destroy User Event(user event=w18, error in=w1) -> (error out=w23:errorcluster)
  n113 = call <vilib>:"Simple Error Handler.vi"("error in (no error)"=w23) -> ("error out"=w11:errorcluster)  [unwired: 4 in, 4 out]
  n114 = control-ref of="This VI"() -> (w10:refnum<vi>)
  n115 = invoke class="VI" method="FP.Close"(reference=w10, error in=w11) -> (reference out=w8:refnum<vi>, error out=w9:errorcluster)  [unwired: 1 in, 1 out]
  n116 = Close Reference(reference=w8, error in (no error)=w9) -> ()  [unwired: 1 out]
